vi "FT_status to error.vi"(8 "error in":errorcluster, 11 "FT_Status":u32) -> (0 "error out":errorcluster)   [LabVIEW 2019]
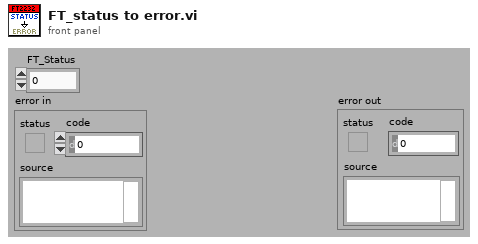
[diagram p1: front panel]
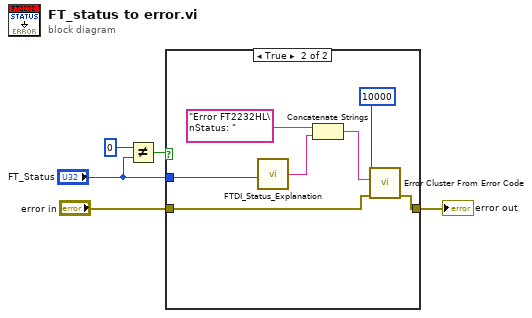
[diagram p0: block diagram]
diagram:
  n1 = Not Equal?(x=u32 0, y="FT_Status") -> (x != y?=w1:bool)
  n2 = case shown="True" w1 {
    tunnel: "error in" -> [w6 w9]
    tunnel: [w6 w8] -> w4
    tunnel: "FT_Status" -> [_ w7]
    frame False {
    }
    frame True {
      n3 = call "FTDI_Status_Explanation.vi"("FT_Status"=w7) -> ("Status String"=w11:string)
      n4 = Concatenate Strings("Error FT2232HL\nStatus: ", w11) -> (w10:string)
      n5 = call <vilib>:"Error Cluster From Error Code.vi"("error in (no error)"=w9, "error message (\"\")"=w10, "error code (0)"=10000 ("error code (no error:0)")) -> ("error out"=w8:errorcluster)  [unwired: 1 in, 5 out]
    }
  }
  "error out" <- w4
